vi "PulsedstressV_inputs.vi"() -> ()   [LabVIEW 2009]
panel:
  out "Actual Stress Time (s)":dbl format="%.4f"
  out "Pulse OFF width errors":string
  out "Pulse ON width errors":string
  out "Period errors":string
  out "Stress time errors":string
  out "SPA single/double":string
  out "SPA Vextra_stop":dbl format="%.3f"
  out "SPA pulse width (not actual)":dbl format="%.4f"
  out "SPA Period":dbl format="%.4f"
  in  "Desired Stress time (s)":dbl format="%.4f"
  in  "Desired Pulse ON width (s)":dbl format="%.4f"
  in  "Desired Period (s)":dbl format="%.4f"
  # "Desired pulse parameters (INPUTS)"
  # "(OUTPUTS) Values for pulsedVstress line in textcontrol.vi"
  # "ERRORS (must be corrected before running pulsed stress!)"
  # "WARNING:\nIn the pulsedstressV program in textcontrol.vi, the following variables \nare hard coded, and any changes to them in the text control screen or \ncommand lines (e.g. itime, pulsed ON, etc.)  will be ignored \nduring and after the pulsed stress step, until they are reset using the\ncomments (itime, pulsed ON, etc.)\n   integration = set at SHORT\n   D/G/SMU4 compliance = set at 10 mA\n   G/SMU4 range = fixed at 1 mA\n   S range = fixed at 10 mA\n   D range = limited auto at 10 uA"
  # "How to do pulsed stress following the method \nof Salleo et al, APL 86 263505 (2005):\n(1) Due to our SPA configuration, only limited ranges are available for pulse period, pulse width, and total stress time. Input your desired parameters into this program, adjust them to eliminate any errors, and then note the output values on the right hand side.\n(2) Write a script file to be run in \"text control.vi\".  The first line should be the stress. For DC voltage stress, use\n     sample Vg Vd NumSamples Time(s) SampleInterval(s)\nwhere SampleInterval(s) is usually 0.004, NumSamples is high (typically 3000, but must be less than Time/SampleInterval), and the length of the bias stress time is Time(s). Note that NumSamples and SampleInterval(s) do not affect the bias stress itself - they only change the recording of data.    \\/\\/\\/\\/...continued below...\\/\\/\\/\\/\n\nFor pulsed bias stress, use\n     pulsedstressV [s|d] VEstop VgON VgOFF Period(s) PulseONwidth(s) Vd\nwhere s/d, VEstop, Period(s) and PulseONwidth(s) are all given by the outputs of THIS program.\n\nFor the recovery section, if you want the currents to be measured using pulsed gate voltages, then issue (once) the command\n      pulsed on PulsePeriod(sec) PulsedGateOFFVoltage PulseONWidth(sec)\nIf a short DC bias is acceptable, then set the integration time as desired on the screen - no further command is needed.\nIn the script, add the following set of commands, repeated as many times as needed:\n      wait 7500\n      transfer s VG VG 0 VD VD 0\n      wait 7500\n      transfer s VG VG 0 VD VD 0\n      wait 7500\n      transfer s VG VG 0 VD VD 0     ...\nThe time in the wait statement is in milliseconds, and should be approx. 2500 ms less than the desired spacing between recovery current measurements (here 10 sec). Note that this uses a transfer \"sweep\" at a single VGS, VDS bias point to measure the recovery current. Repeat these two lines as many times as you like (can be thousands!) to measure the recovery over long periods.\n\n(3) Before running, in the Panels Controls 2 box, set the Text/Graph to \"text\" (so that the green light is OFF). This must be done or the recovery measurements will not work. Also set D/G compliance to 0.01 A, integration to short and D/G/S range to Limited 10uA (These last two settings will affect the time it takes to make each non-pulsed recovery measurement, which generally you want to be as short as possible.)\n\nBecause of the complexity, I recommend doing an abbreviated trial run on a test TFT before trying your precious devices!"
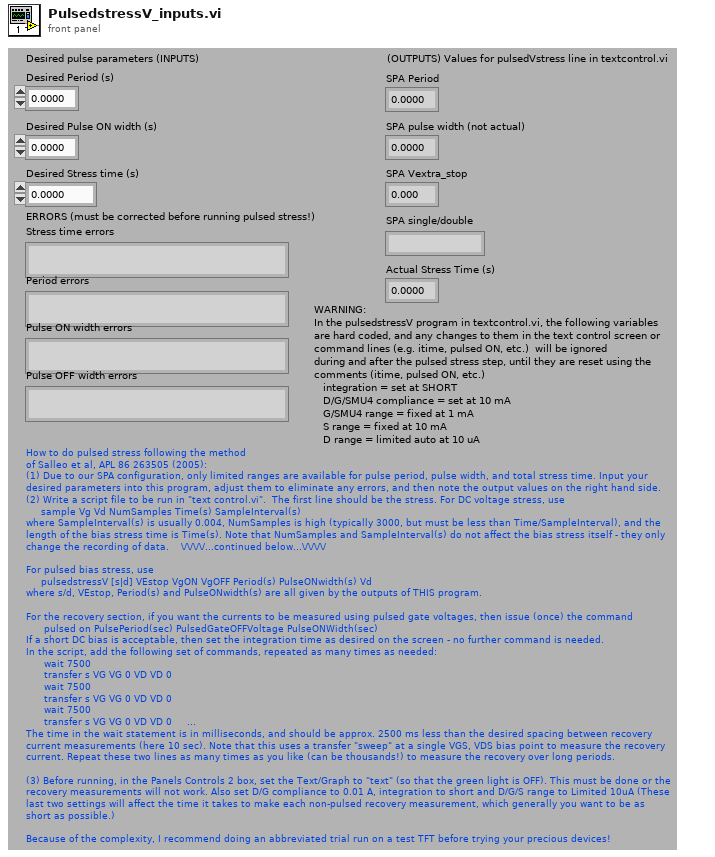
[diagram p1: front panel]
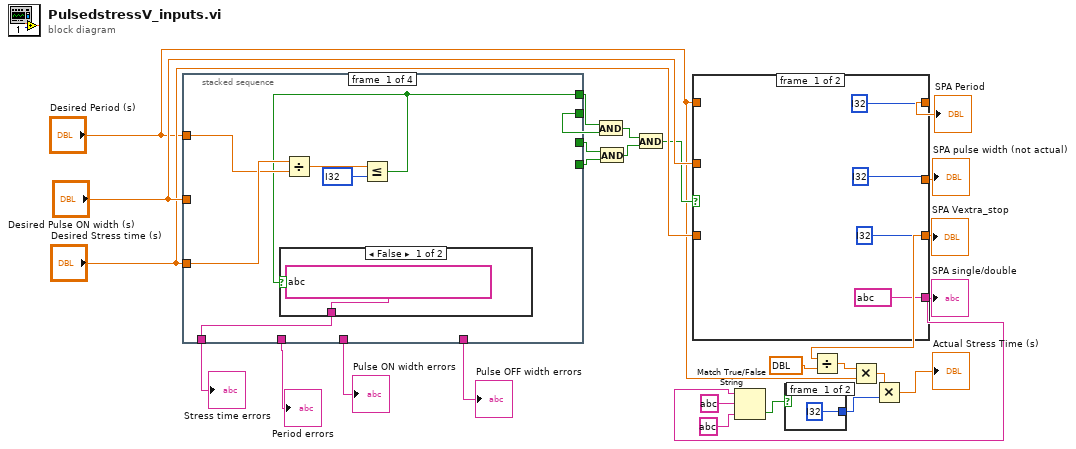
[diagram p0: block diagram]
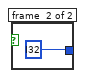
[diagram p2: hidden frame]
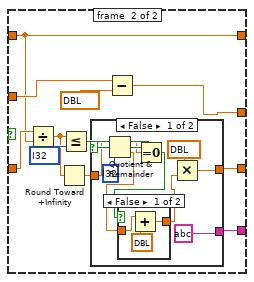
[diagram p3: hidden frame]
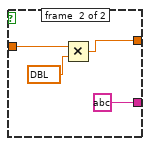
[diagram p5: hidden frame]
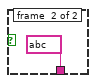
[diagram p6: hidden frame]
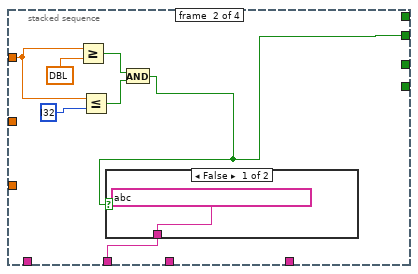
[diagram p7: hidden frame]
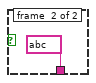
[diagram p8: hidden frame]
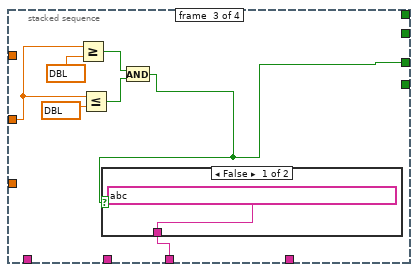
[diagram p9: hidden frame]
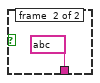
[diagram p10: hidden frame]
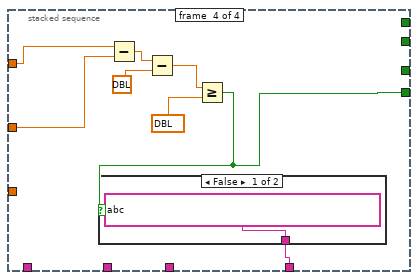
[diagram p11: hidden frame]
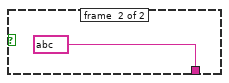
[diagram p12: hidden frame]
diagram:
  n1 = stacked-sequence {
    tunnel: "Desired Period (s)" -> [w31 w41 _ w59]
    tunnel: "Desired Pulse ON width (s)" -> [_ _ w44 w58]
    tunnel: "Desired Stress time (s)" -> [w32 _ _ _]
    tunnel: [w28 _ _ _] -> w25
    tunnel: [w27 _ _ _] -> w26
    tunnel: [_ w36 _ _] -> w24
    tunnel: [_ w35 _ _] -> w23
    tunnel: [_ _ w46 _] -> w20
    tunnel: [_ _ w45 _] -> w22
    tunnel: [_ _ _ w54] -> w21
    tunnel: [_ _ _ w53] -> w17
    frame #0 {
      n2 = Divide(x=w32, y=w31) -> (x/y=w29:dbl)
      n3 = Less Or Equal?(x=w29, y=i32 ?) -> (x <= y?=w28:bool)
      n4 = case shown="False" w28 {
        tunnel: [string ? string ?] -> w27
        frame #0 {
        }
        frame #1 {
        }
      }
    }
    frame #1 {
      n5 = Greater Or Equal?(x=w41, y=dbl ?) -> (x >= y?=w38:bool)
      n6 = Less Or Equal?(x=w41, y=i32 ?) -> (x <= y?=w37:bool)
      n7 = And(x=w38, y=w37) -> (x .and. y?=w36:bool)
      n8 = case shown="False" w36 {
        tunnel: [string ? string ?] -> w35
        frame #0 {
        }
        frame #1 {
        }
      }
    }
    frame #2 {
      n9 = Greater Or Equal?(x=w44, y=dbl ?) -> (x >= y?=w48:bool)
      n10 = Less Or Equal?(x=w44, y=dbl ?) -> (x <= y?=w47:bool)
      n11 = And(x=w48, y=w47) -> (x .and. y?=w46:bool)
      n12 = case shown="False" w46 {
        tunnel: [string ? string ?] -> w45
        frame #0 {
        }
        frame #1 {
        }
      }
    }
    frame #3 {
      n13 = Subtract(x=w59, y=w58) -> (x-y=w57:dbl)
      n14 = Subtract(x=w57, y=dbl ?) -> (x-y=w55:dbl)
      n15 = Greater Or Equal?(x=w55, y=dbl ?) -> (x >= y?=w54:bool)
      n16 = case shown="False" w54 {
        tunnel: [string ? string ?] -> w53
        frame #0 {
        }
        frame #1 {
        }
      }
    }
  }
  "Stress time errors" <- w26
  "Period errors" <- w23
  "Pulse ON width errors" <- w22
  "Pulse OFF width errors" <- w17
  n17 = And(x=w25, y=w24) -> (x .and. y?=w19:bool)
  n18 = And(x=w20, y=w21) -> (x .and. y?=w18:bool)
  n19 = And(x=w19, y=w18) -> (x .and. y?=w12:bool)
  n20 = case shown="True" w12 {
    tunnel: "Desired Period (s)" -> [_ w67]
    tunnel: [i32 ? w67] -> w16
    tunnel: "Desired Pulse ON width (s)" -> [_ w77]
    tunnel: "Desired Stress time (s)" -> [_ w74]
    tunnel: [i32 ? w76] -> w13
    tunnel: [string ? w71] -> w3
    tunnel: [i32 ? w70] -> w11
    frame #0 {
    }
    frame #1 {
      n21 = Divide(x=w74, y=w67) -> (x/y=w69:dbl)
      n22 = Round Toward +Infinity(x=w69) -> (ceil(x): smallest int >= x=w68:dbl)
      n23 = Less Or Equal?(x=w69, y=i32 ?) -> (x <= y?=w72:bool)
      n24 = case shown="False" w72 {
        tunnel: [string ? string ?] -> w71
        tunnel: [w81 w92] -> w70
        tunnel: w68 -> [w85 w91]
        frame #0 {
          n25 = Quotient & Remainder(x=w85, y=i32 ?) -> (x-y*floor(x/y)=w79:dbl, floor(x/y)=w78:dbl)
          n26 = Equal To 0?(x=w79) -> (x = 0?=w83:bool)
          n27 = case shown="False" w83 {
            tunnel: [w89 w90] -> w80
            tunnel: w78 -> [w88 w90]
            frame #0 {
              n28 = Add(x=w88, y=dbl ?) -> (x+y=w89:dbl)
            }
            frame #1 {
            }
          }
          n29 = Multiply(x=dbl ?, y=w80) -> (x*y=w81:dbl)
        }
        frame #1 {
          n30 = Multiply(x=w91, y=dbl ?) -> (x*y=w92:dbl)
        }
      }
      n31 = Subtract(x=w77, y=dbl ?) -> (x-y=w76:dbl)
    }
  }
  "SPA Period" <- w16
  "SPA pulse width (not actual)" <- w13
  "SPA Vextra_stop" <- w11
  "SPA single/double" <- w3
  n32 = Match True/False String(2:string ?, 3:string ?, 4:w3) -> (0:w4:bool)  [unwired: 1 out]
  n33 = case shown="True" w4 {
    tunnel: [i32 ? i32 ?] -> w5
    frame #0 {
    }
    frame #1 {
    }
  }
  n34 = Divide(x=w11, y=dbl ?) -> (x/y=w9:dbl)
  n35 = Multiply(x=w9, y="Desired Period (s)") -> (x*y=w7:dbl)
  n36 = Multiply(x=w7, y=w5) -> (x*y=→"Actual Stress Time (s)":dbl)
